vi "Send Identification.vi"(0 "RS232 Port In":refnum<visa-resource-name>="COM12", 1 "Sensor Address In":string="0", 3 "Initialize/Close?":bool, 7 "Error In (No Error)":errorcluster) -> (20 "RS232 Port Out":refnum<visa-resource-name>, 21 "Address Out":string, 22 "SDI-12 Compatibility Number":dbl, 23 "Company Name":string, 24 "Sensor Model Number":string, 25 "Sensor Version":string, 26 "Serial Number/MISC":string, 27 "Error Out":errorcluster)   [LabVIEW 2016]
doc: "Sends an SDI-12 Send Identification Command, and returns the various attributes from the sensor's response.\n\nThe total size by the sensor must be 22-35 in size (inclusive), or this VI will return an error."
uses:
  SDI-12.lvlib
panel:
  out "length":i32
  out "Serial Settings:Number of Bytes at Serial Port":u32
  # "(c) 2008 National Instruments.  ALL RIGHTS RESERVED."
  # "The following are required,\nor are optional, for the sensors\nto respond with:"
  # "Length:"
  # "REQUIRED:"
  # "1 FIXED"
  # "REQUIRED:"
  # "2 FIXED"
  # "REQUIRED:"
  # "8 FIXED"
  # "REQUIRED:"
  # "6 FIXED"
  # "REQUIRED:"
  # "3 FIXED"
  # "OPTIONAL:"
  # "1-13 Inclusive Variable"
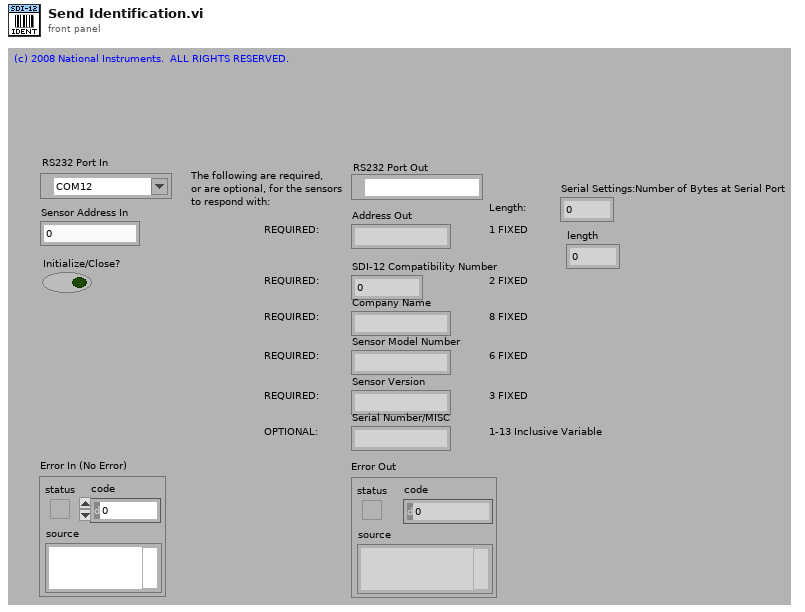
[diagram p1: front panel]
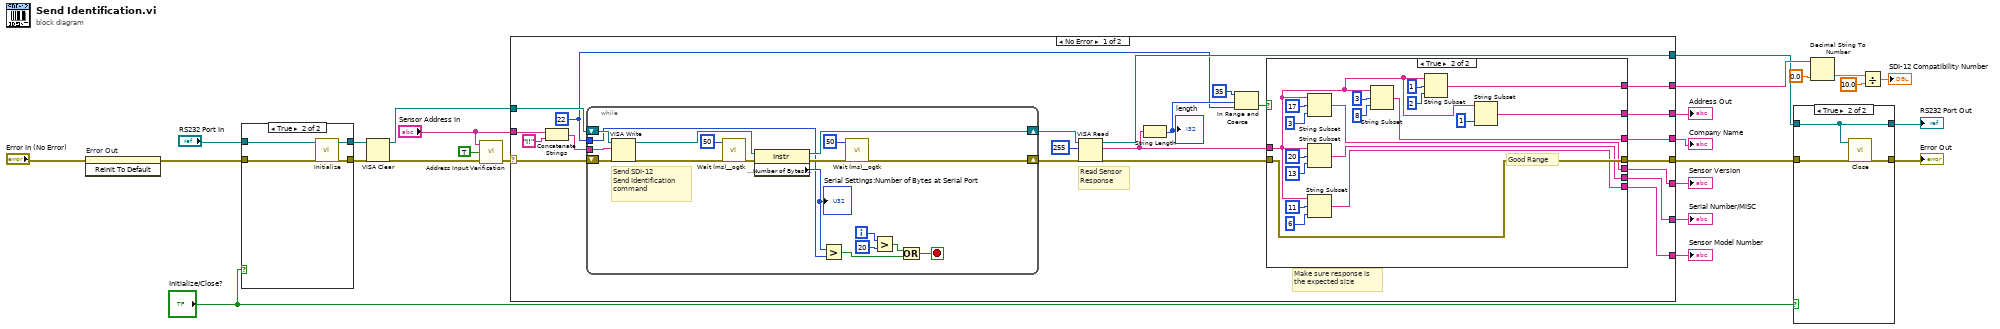
[diagram p0: block diagram]
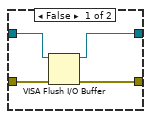
[diagram p2: hidden frame]
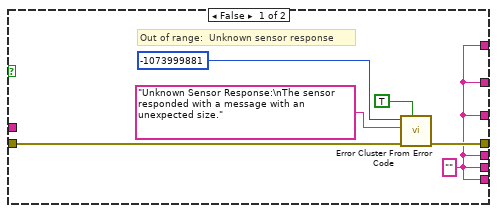
[diagram p4: hidden frame]
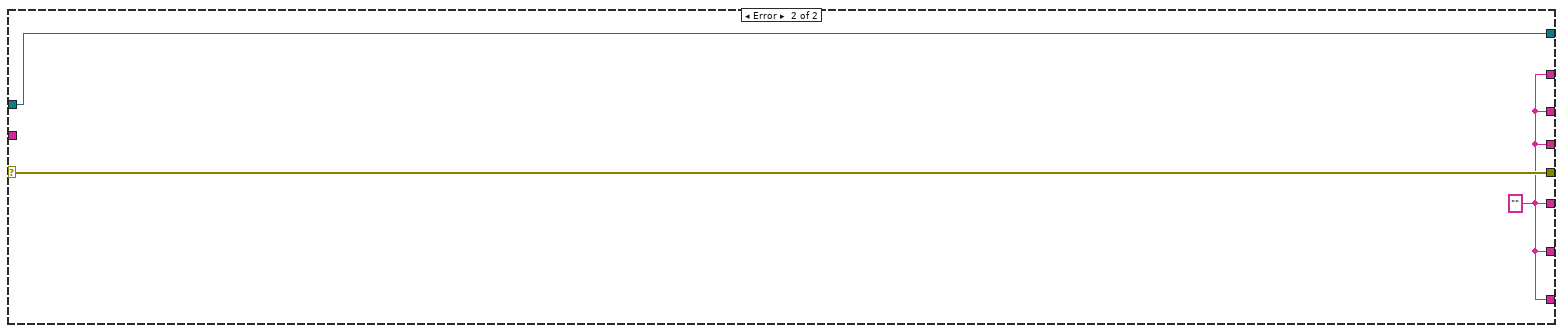
[diagram p5: hidden frame]
diagram:
  n1 = invoke on="Error Out" class="Clust (strict)" method="Reinit To Default"(error in="Error In (No Error)") -> (error out=w9:errorcluster)  [unwired: 2 in, 2 out]
  n2 = case shown="True" "Initialize/Close?" {
    tunnel: w9 -> [w27 w31]
    tunnel: [w27 w30] -> w8
    tunnel: "RS232 Port In" -> [w26 w29]
    tunnel: [w26 w28] -> w6
    frame False {
    }
    frame True {
      n3 = call "Initialize.vi"("Error In (No Error)"=w31, "RS232 Port In"=w29) -> ("Error Out"=w30:errorcluster, "RS232 Port Out"=w28:refnum<visa-resource-name>)  [unwired: 8 in]
    }
  }
  n4 = VISA Clear(VISA resource name=w6, error in (no error)=w8) -> (VISA resource name out=w10:refnum<visa-resource-name>, error out=w11:errorcluster)
  n5 = call "Address Input Verification.vi"("Error In (No Error)"=w11, "Error if Bad? (True)"=TRUE ("error if bad? (True)"), "Sensor Address In (a)"="Sensor Address In") -> ("Error Out"=w25:errorcluster)  [unwired: 1 in, 1 out]
  n6 = case shown="No Error" w25 {
    selector: w25 -> [w52 w99]
    tunnel: [w41 w99] -> w5
    tunnel: "Sensor Address In" -> [w51 _]
    tunnel: w10 -> [w48 w98]
    tunnel: [w47 w98] -> w3
    tunnel: [w40 w97] -> w22
    tunnel: [w39 w97] -> w21
    tunnel: [w38 w97] -> w20
    tunnel: [w37 w97] -> w19
    tunnel: [w36 w97] -> w17
    tunnel: [w35 w97] -> w18
    frame No Error {
      w32 = 22 ("lower limit")
      # "Make sure response is\nthe expected size"
      # "Read Sensor\nResponse"
      n7 = Concatenate Strings(w51, "I!" ("write buffer")) -> (w49:string)
      n8 = while {
        tunnel: w49 -> [w69]
        shift-right: [w58] -> w33
        shift-left: w52 -> [w70]
        shift-right: [w67] -> w34
        shift-left: w48 -> [w55]
        tunnel: w32 -> [w54]
        i -> [w59]
        stop <- w60 stop-if-true
        # "Send SDI-12 \nSend Identification \ncommand"
        n9 = VISA Write(VISA resource name=w55, write buffer=w69, error in (no error)=w70) -> (VISA resource name out=w68:refnum<visa-resource-name>, error out=w71:errorcluster)  [unwired: 1 out]
        n10 = call "Wait (ms)__ogtk.vi"("error in (no error)"=w71, "milliseconds to wait"=u32 50) -> ("error out"=w64:errorcluster)  [unwired: 8 in, 1 out]
        n11 = property class="Instr"(reference=w68, error in=w64) -> (reference out=w67:refnum<visa-resource-name>, error out=w66:errorcluster, "Serial Settings:Number of Bytes at Serial Port"=w56:u32)
        "Serial Settings:Number of Bytes at Serial Port" <- w56
        n12 = Greater?(x=w56, y=w54) -> (0:w63:bool)
        n13 = call "Wait (ms)__ogtk.vi"("error in (no error)"=w66, "milliseconds to wait"=u32 50) -> ("error out"=w58:errorcluster)  [unwired: 8 in, 1 out]
        n14 = Greater?(x=w59, y=20) -> (0:w62:bool)
        n15 = Or(x=w62, y=w63) -> (x .or. y?=w60:bool)
      }
      n16 = VISA Read(VISA resource name=w34, byte count=u32 255, error in (no error)=w33) -> (VISA resource name out=w47:refnum<visa-resource-name>, read buffer=w43:string, error out=w44:errorcluster)  [unwired: 1 out]
      n17 = String Length(string=w43) -> (length=w45:i32)
      "length" <- w45
      n18 = In Range and Coerce(upper limit=35, x=w45, lower limit=w32) -> (In Range?=w42:bool)  [unwired: 1 out]
      n19 = case shown="True" w42 {
        tunnel: w44 -> [w73 w84]
        tunnel: [w74 w84] -> w41
        tunnel: w43 -> [_ w90]
        tunnel: [w72 w83] -> w40
        tunnel: [w72 w82] -> w39
        tunnel: [w72 w81] -> w38
        tunnel: [w72 w80] -> w37
        tunnel: [w72 w79] -> w36
        tunnel: [w72 w78] -> w35
        frame False {
          w72 = "" ("read buffer")
          # "Out of range:  Unknown sensor response"
          n20 = call <vilib>:"Error Cluster From Error Code.vi"("show call chain? (False)"=TRUE, "error in (no error)"=w73, "error message (\"\")"="Unknown Sensor Response:\nThe sensor responded with a message with an unexpected size." ("error message (\"\")"), "error code (0)"=-1073999881) -> ("error out"=w74:errorcluster)  [unwired: 5 in]
        }
        frame True {
          # "Good Range"
          n21 = String Subset(string=w90, offset (0)=17, length (rest)=3 ("length (rest)")) -> (substring=w82:string)
          n22 = String Subset(string=w90, offset (0)=20, length (rest)=13 ("length (rest)")) -> (substring=w83:string)
          n23 = String Subset(string=w90, offset (0)=11, length (rest)=6 ("length (rest)")) -> (substring=w81:string)
          n24 = String Subset(string=w90, offset (0)=3, length (rest)=8 ("length (rest)")) -> (substring=w80:string)
          n25 = String Subset(string=w90, offset (0)=1, length (rest)=2 ("length (rest)")) -> (substring=w79:string)
          n26 = String Subset(string=w90, length (rest)=1 ("length (rest)")) -> (substring=w78:string)  [unwired: 1 in]
        }
      }
    }
    frame Error {
      w97 = "" ("read buffer")
    }
  }
  "Serial Number/MISC" <- w22
  "Sensor Version" <- w21
  "Sensor Model Number" <- w20
  "Company Name" <- w19
  "Address Out" <- w18
  n27 = case shown="True" "Initialize/Close?" {
    tunnel: w5 -> [w103 w106]
    tunnel: [w102 w105] -> w4
    tunnel: w3 -> [w101 w104]
    tunnel: [w100 w104] -> w1
    frame False {
      n28 = VISA Flush I/O Buffer(VISA resource name=w101, error in (no error)=w103) -> (VISA resource name out=w100:refnum<visa-resource-name>, error out=w102:errorcluster)  [unwired: 1 in]
    }
    frame True {
      n29 = call "Close.vi"("Error In (No Error)"=w106, "RS232 Port In"=w104) -> ("Error Out"=w105:errorcluster)  [unwired: 9 in]
    }
  }
  "Error Out" <- w4
  "RS232 Port Out" <- w1
  n30 = Decimal String To Number(string=w17, default (0L)=0.0 ("default (0 I32)")) -> (number=w14:dbl)  [unwired: 1 in, 1 out]
  n31 = Divide(x=w14, y=10.0) -> (x/y=→"SDI-12 Compatibility Number":dbl)
